vi "Run.vi"(8 "error in (no error)":errorcluster caption="entrée d'erreur (pas d'erreur)", 9 "X":string[][](array[string]), 10 "Type X":T1(ring), 11 "add_dummy_feature.lvclass":refnum<class "add_dummy_feature.lvclass">) -> (0 "error out":errorcluster caption="sortie d'erreur", 2 "Data":T2, 3 "add_dummy_feature.lvclass":refnum<class "add_dummy_feature.lvclass">)   [LabVIEW 2020, in "add_dummy_feature.lvclass"]
doc: "Returns :\n\n- X : {array, sparse matrix}, shape [n_samples, n_features + 1]\nSame data with dummy feature added as first column."
uses:
  add_dummy_feature.lvclass
  add_dummy_feature.lvclass/add_dummy_feature.ctl
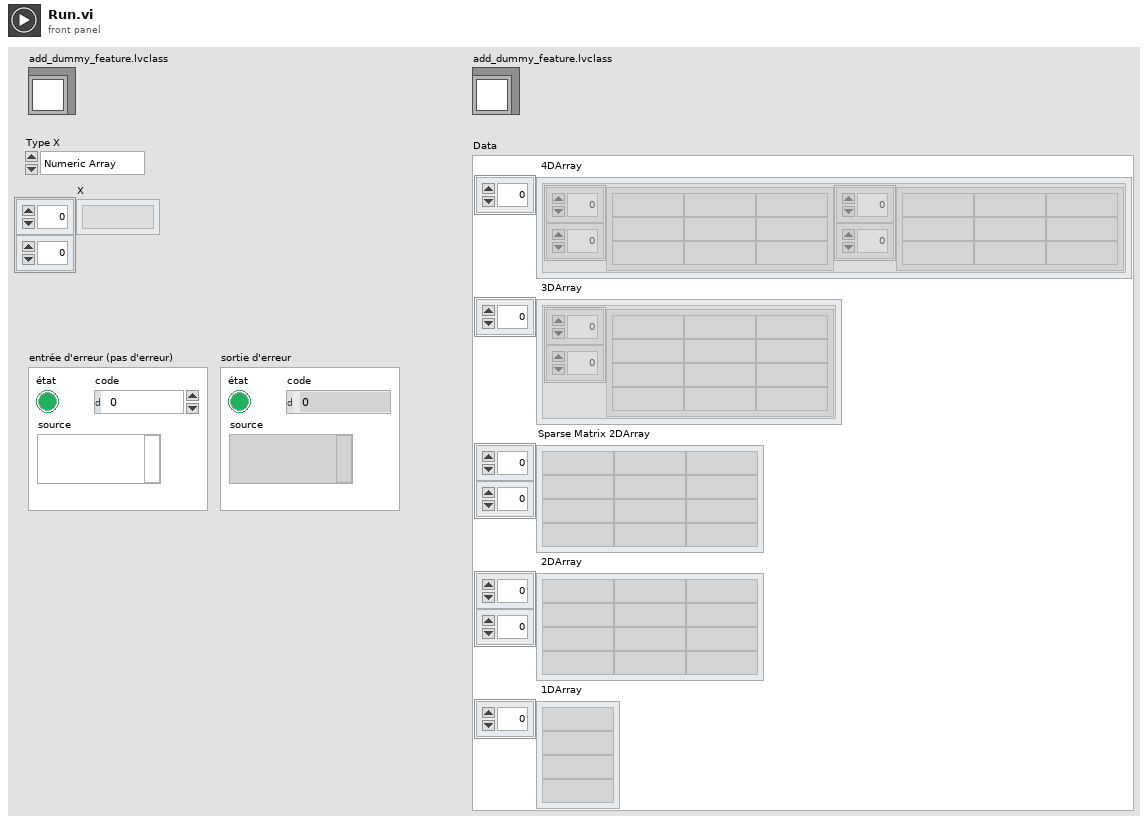
[diagram p1: front panel]
types:
  T1 = enum16{"Numeric Array", "String Array", "Sparse"}
  T2 = cluster{" 4DArray":cluster{"1":string[][], "2":string[][]}[], " 3DArray":cluster{"Tableau":string[][]}[], "Sparse Matrix 2DArray":string[][], " 2DArray":string[][], " 1DArray":string[]}
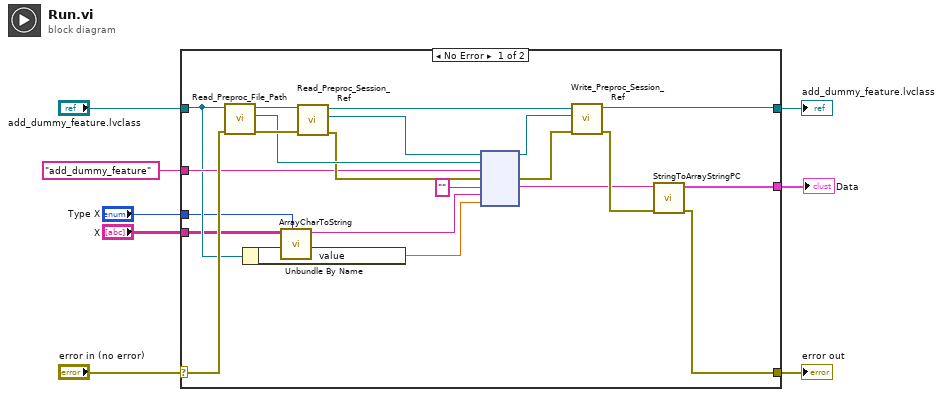
[diagram p0: block diagram]
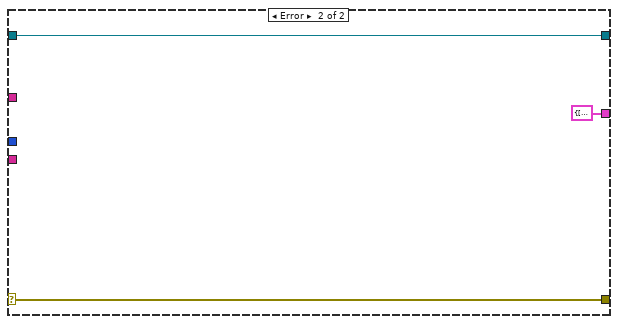
[diagram p2: hidden frame]
diagram:
  n1 = case shown="No Error" "error in (no error)" {
    selector: "error in (no error)" -> [w19 w32]
    tunnel: [w12 w32] -> w7
    tunnel: [w9 w31] -> w5
    tunnel: "add_dummy_feature.lvclass" -> [w17 w31]
    tunnel: "add_dummy_feature" ("Fonction") -> [w18 _]
    tunnel: [w10 T2 {" 4DArray"=[], " 3DArray"=[], "Sparse Matrix 2DArray"=[], " 2DArray"=[], " 1DArray"=[]} ("Data")] -> w1
    tunnel: "X" -> [w15 _]
    tunnel: "Type X" -> [w16 _]
    frame No Error {
      n2 = call-dynamic "Read_Preproc_File_Path.vi"("error in (no error)"=w19, "Python in"=w17) -> ("error out"=w28:errorcluster, "File_Path"=w25:path, "Python out"=w29:refnum<class "add_dummy_feature.lvclass">)  [unwired: 7 in]
      n3 = Unbundle By Name(w17) -> ("value"=w20:dbl)
      n4 = call "ArrayCharToString.vi"("Type"=w16, "TAB"=w15) -> ("Instruction"=w14:string)  [unwired: 9 in]
      n5 = call-dynamic "Read_Preproc_Session_Ref.vi"("error in (no error)"=w28, "Python in"=w29) -> ("error out"=w24:errorcluster, "Session_ref"=w26:refnum<k35>, "Python out"=w27:refnum<class "add_dummy_feature.lvclass">)  [unwired: 7 in]
      n6 = node(w26, w25, w18, w24, "", w14, w20) -> (w22:refnum<k35>, w23:errorcluster, w11:string)  [unwired: 2 in, 2 out]
      n7 = call-dynamic "Write_Preproc_Session_Ref.vi"("error in (no error)"=w23, "Session_ref"=w22, "Python in"=w27) -> ("error out"=w13:errorcluster, "Python out"=w9:refnum<class "add_dummy_feature.lvclass">)  [unwired: 7 in]
      n8 = call "StringToArrayStringPC.vi"("sortie d'erreur"=w13, "Return value"=w11) -> ("sortie d'erreur"=w12:errorcluster, "Data"=w10:T2)  [unwired: 8 in]
    }
    frame Error {
    }
  }
  "error out" <- w7
  "add_dummy_feature.lvclass" <- w5
  "Data" <- w1
